vi "Feedback.vi"() -> ()   [LabVIEW 2020]
panel:
  in  "Number 2":i32
  out "Factorial 2":i32
  out "Factorial":i32
  in  "Number":i32
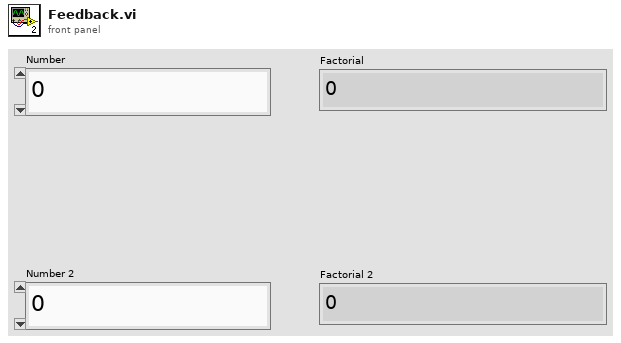
[diagram p1: front panel]
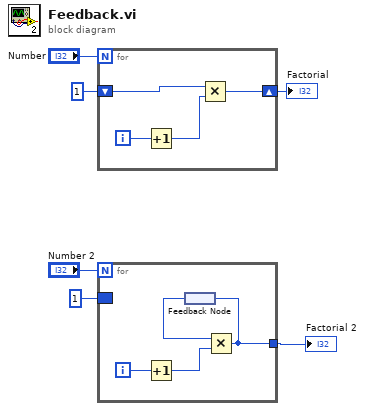
[diagram p0: block diagram]
diagram:
  n1 = for {
    N: "Number" -> [_]
    shift-right: [w7] -> w4
    shift-left: 1 ("x") -> [w8]
    i -> [w10]
    n2 = Increment(x=w10) -> (x+1=w9:i32)
    n3 = Multiply(x=w8, y=w9) -> (x*y=w7:i32)
  }
  "Factorial" <- w4
  n4 = for {
    N: "Number 2" -> [_]
    tunnel: [w11] -> w2
    border: 1 ("x") -> [_]
    i -> [w14]
    n5 = Increment(x=w14) -> (x+1=w13:i32)
    n6 = feedback #1() -> (w12:i32)
    n7 = Multiply(x=w12, y=w13) -> (x*y=w11:i32)
    n8 = feedback-in #1(w11) -> ()
  }
  "Factorial 2" <- w2
